vi "FTW_AppLauncher-Core_Process.vi"(0 "FTW Actor Instance Configuration":string="{\n  \"Identity\": \"ActorName\",\n  \"InboxAddress\": \"inproc://*\",\n  \"LoggerAddress\": \"\",\n  \"DebugEnableInboxLogging\": false,\n  \"DebugEnableJobLogging\": false,\n  \"LauncherAddress\": \"\",\n  \"My Data\": false,\n  \"Publisher URI\": \"inproc://*\",\n  \"Subscriber URIs\": \"\",\n  \"Refresh Period\": 2\n}", 11 "ErrorIn":errorcluster) -> (15 "Error":errorcluster)   [LabVIEW 2013, in "FTW-AppLauncher-Core.lvclass"]
uses:
  FTW-AppLauncher-Core.lvclass
  source/actor/Message/Base/FTW-Message.lvclass
  FTW-AppLauncher-Core.lvclass/FTW-AppLauncher-Core.ctl
  source/actor/Instance/FTW-ActorInstance.lvclass/FTW-ActorInstance.ctl
  source/actor/JobSequencer/FTW-SEQ-Current.vi
  source/actor/Instance/FTW-ActorInstance.lvclass
  source/actor/Message/Request/FTW-Message-IncomingRequest.lvclass
panel:
  out "Status":string
  # "shows the border of the run-time window\nthe orange box will not show"
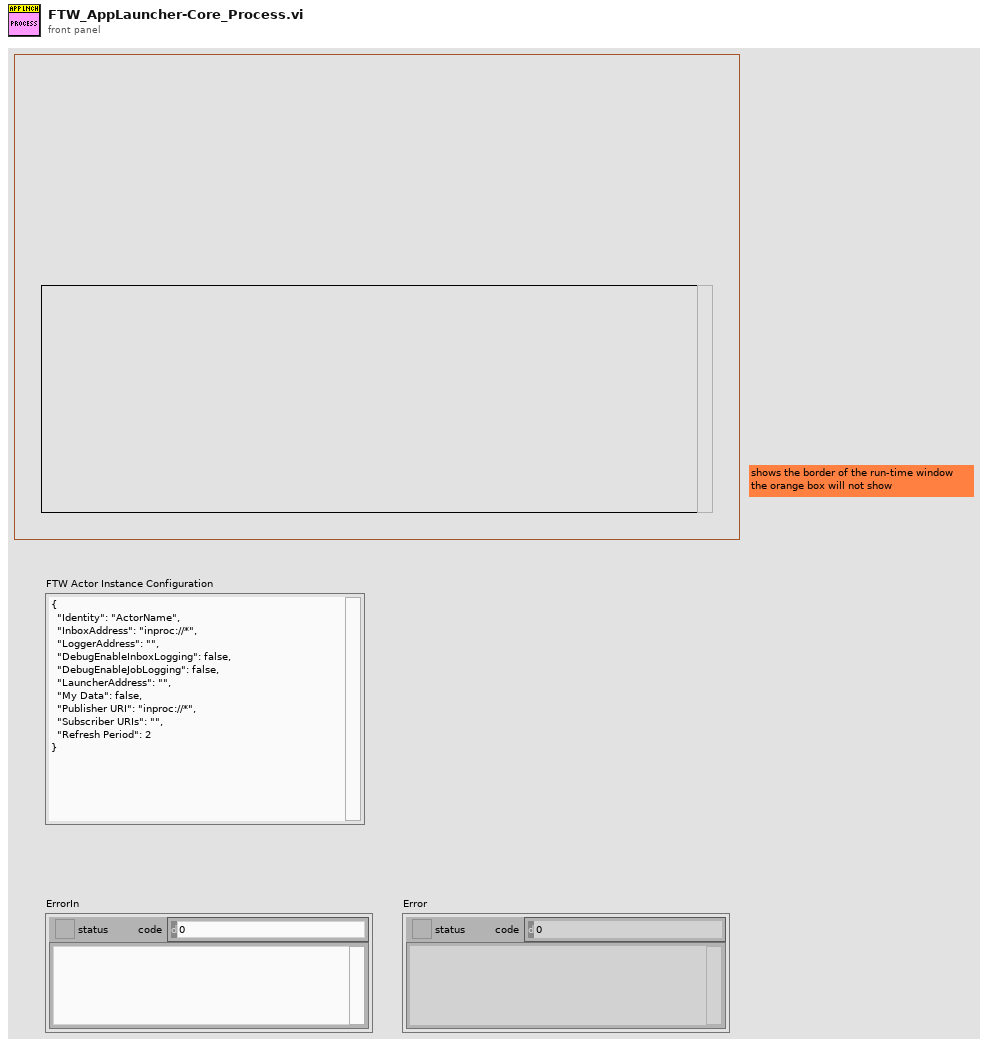
[diagram p1: front panel]
types:
  T1 = cluster{"Incoming Requests":refnum<event-registration>, "Local Messages":refnum<event-registration>, "Subscriber Registration":refnum<event-registration>}
  T2 = cluster{"Identity":string, "Instance Inbox Address":string}
  T3 = cluster{"String":string, "LabVIEW String":string}
  T4 = cluster{"String":string, "LabVIEW String":string}[]
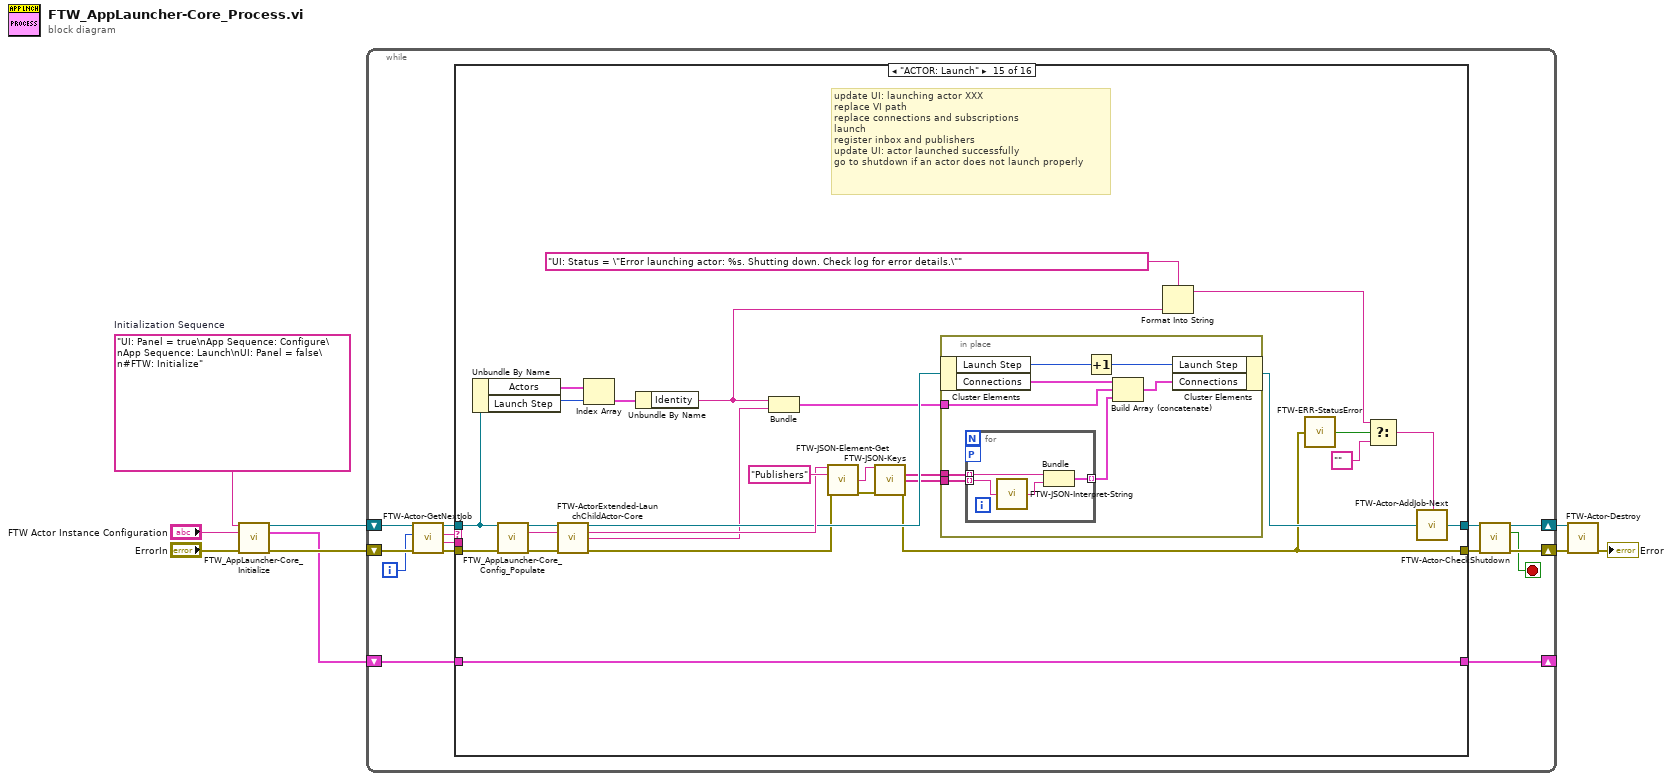
[diagram p0: block diagram]
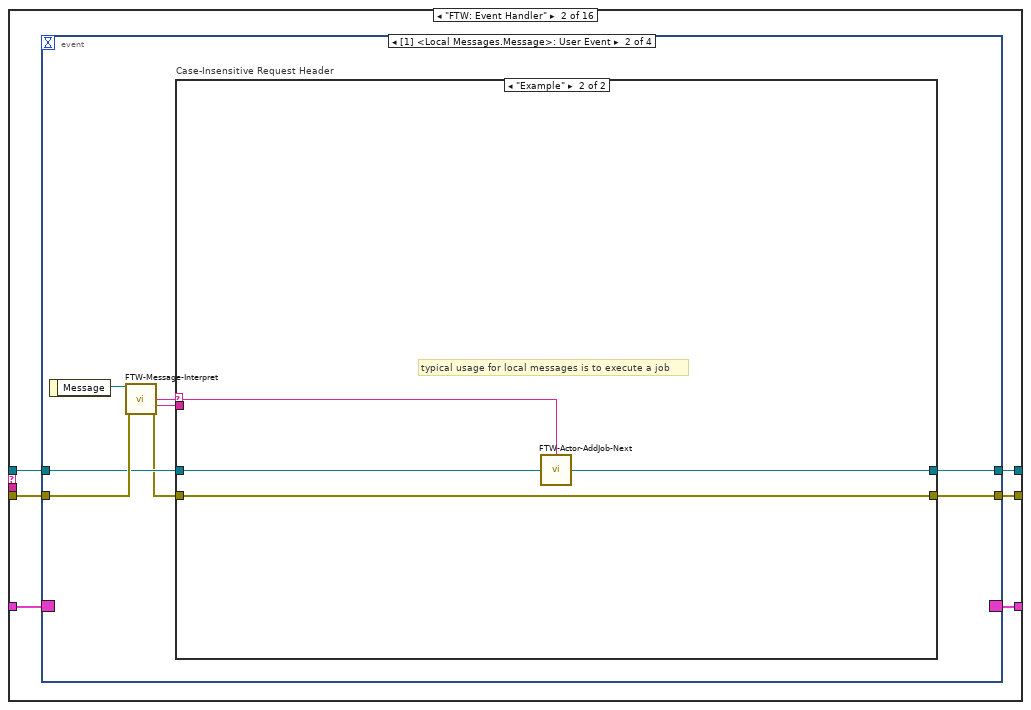
[diagram p3: hidden frame]
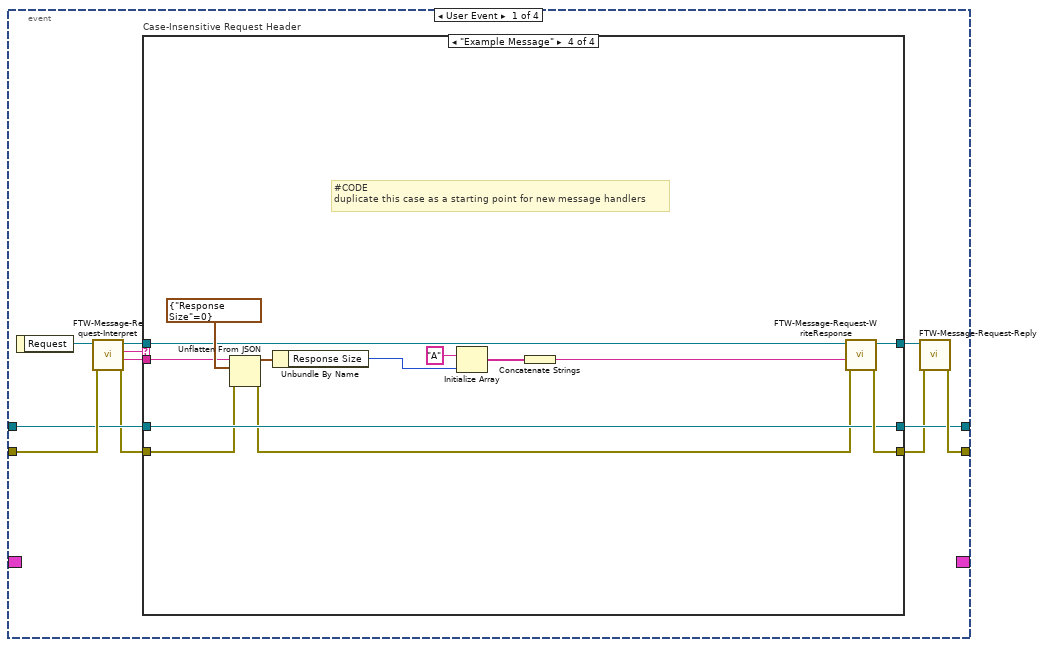
[diagram p4: hidden frame]
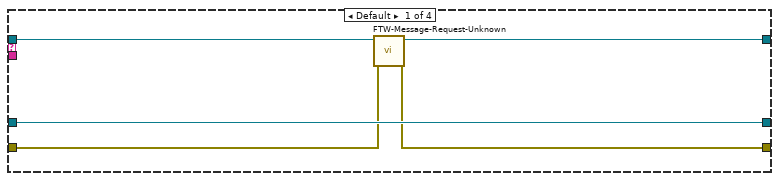
[diagram p5: hidden frame]
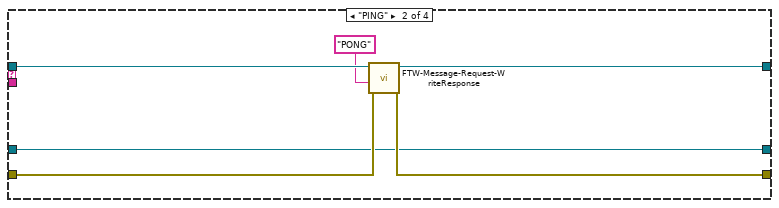
[diagram p6: hidden frame]
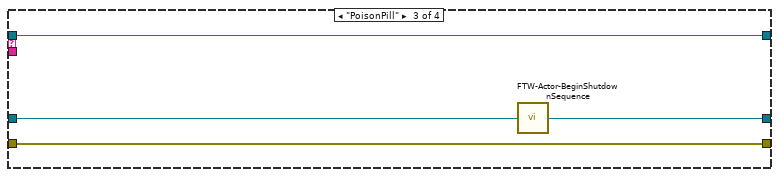
[diagram p7: hidden frame]
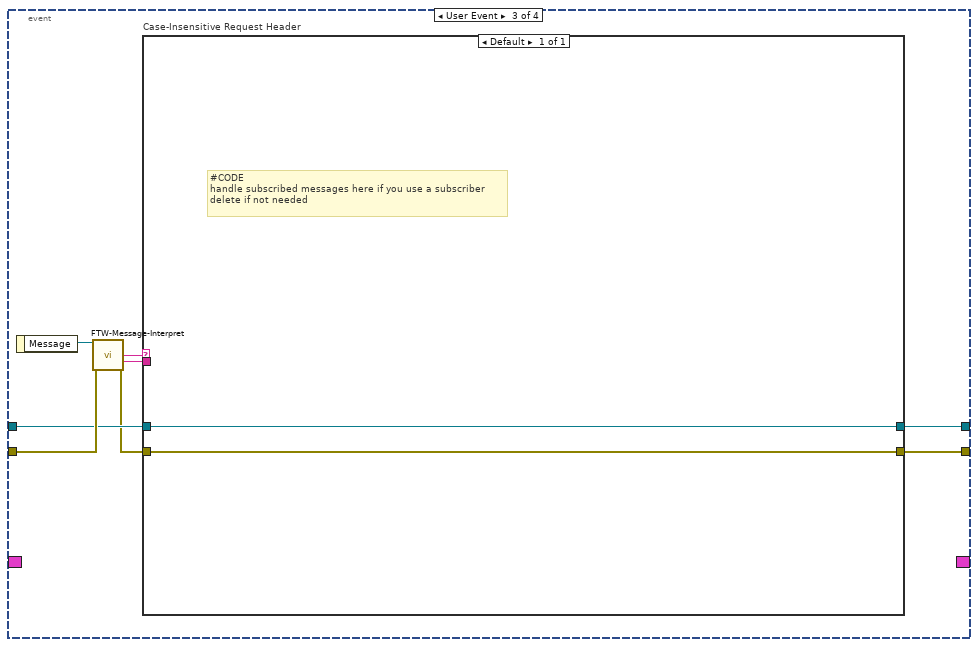
[diagram p9: hidden frame]
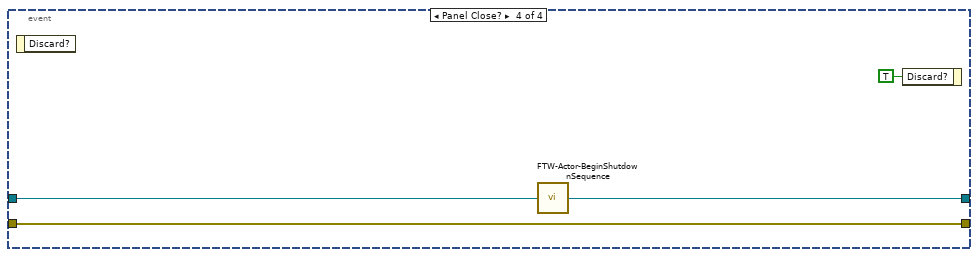
[diagram p10: hidden frame]
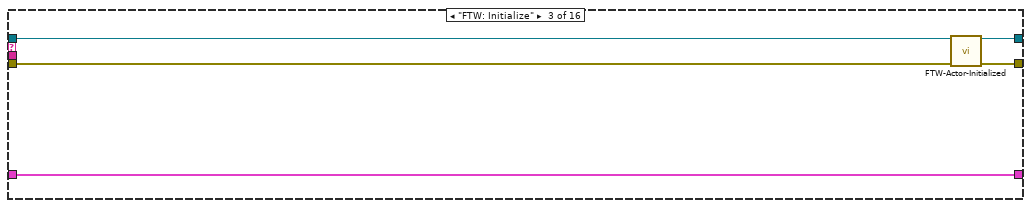
[diagram p11: hidden frame]
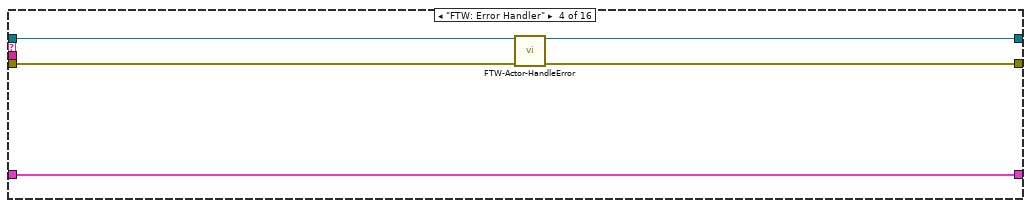
[diagram p12: hidden frame]
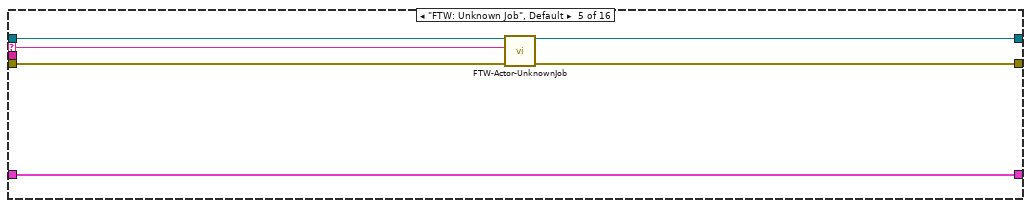
[diagram p13: hidden frame]
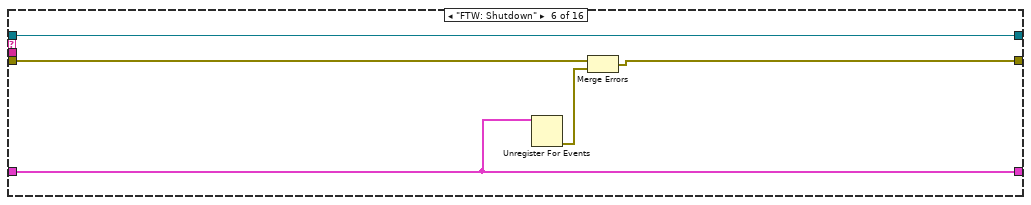
[diagram p14: hidden frame]
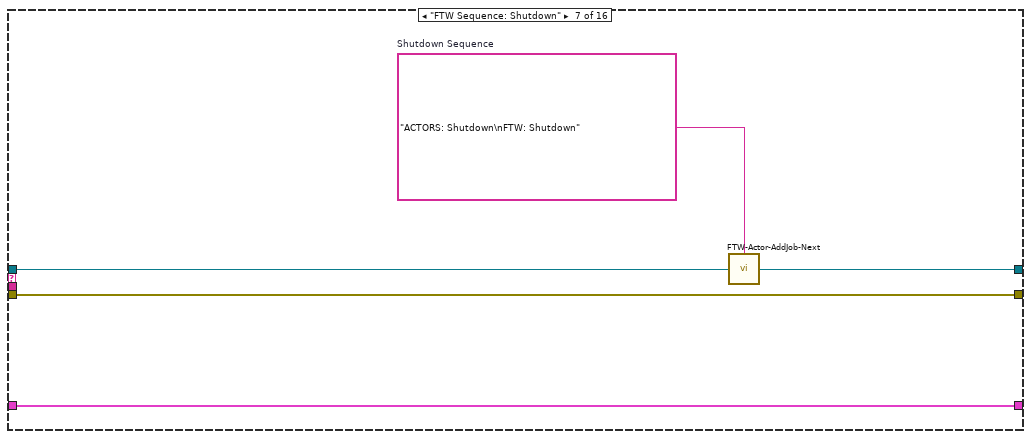
[diagram p15: hidden frame]
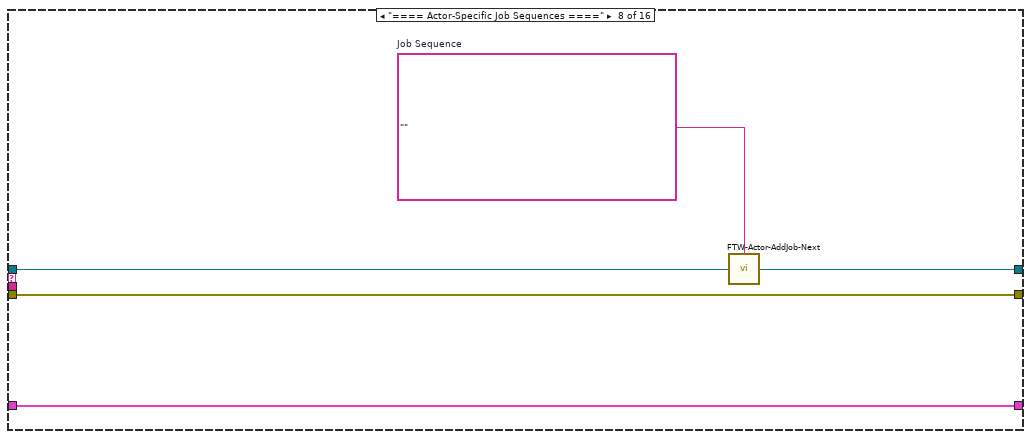
[diagram p16: hidden frame]
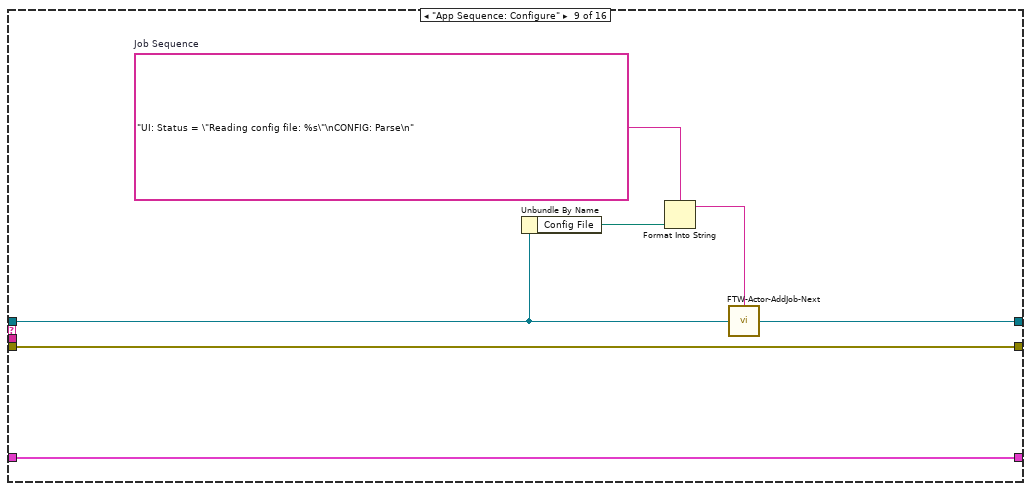
[diagram p17: hidden frame]
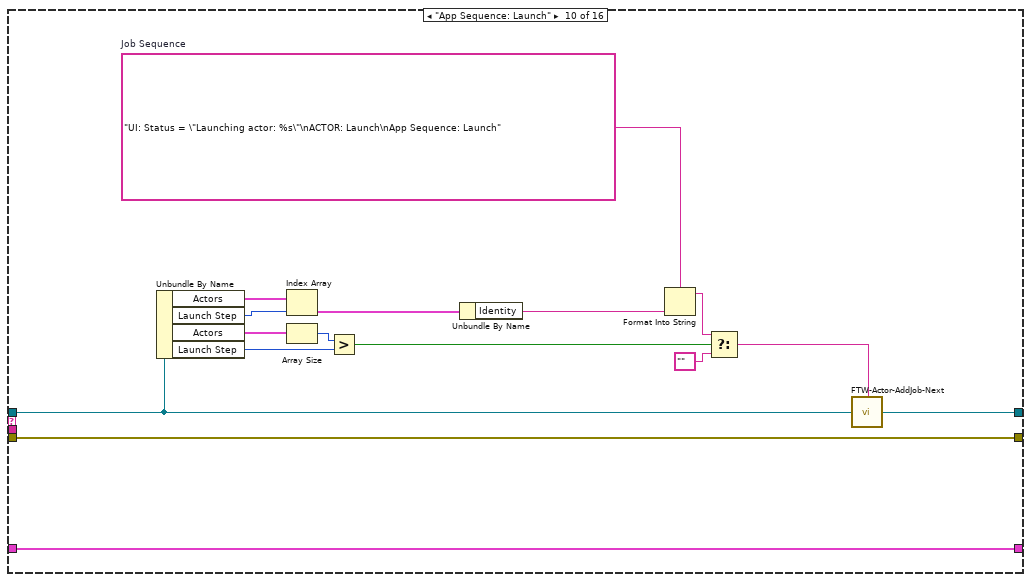
[diagram p18: hidden frame]
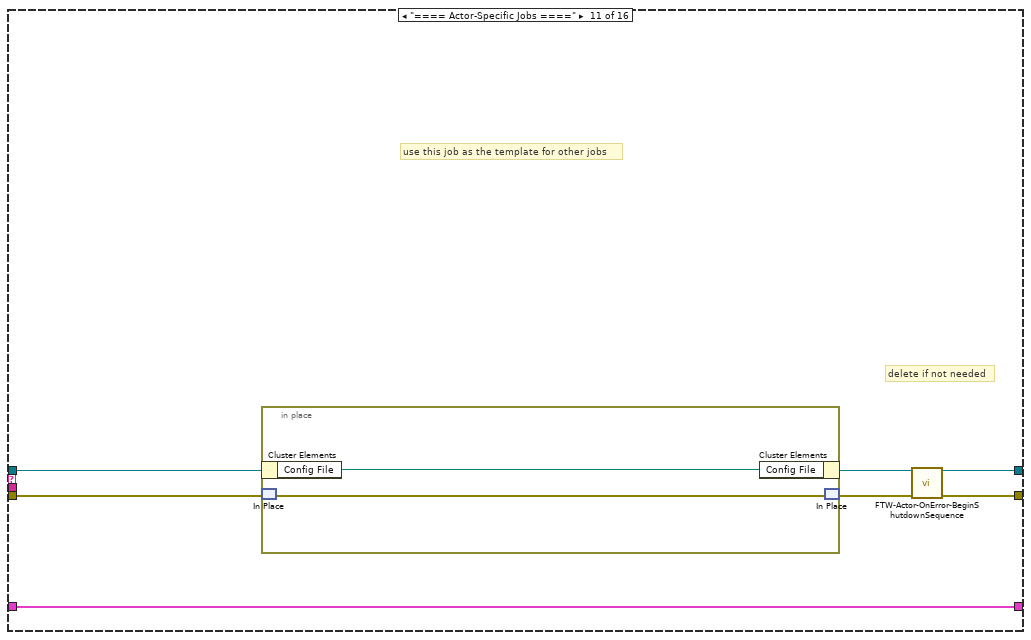
[diagram p19: hidden frame]
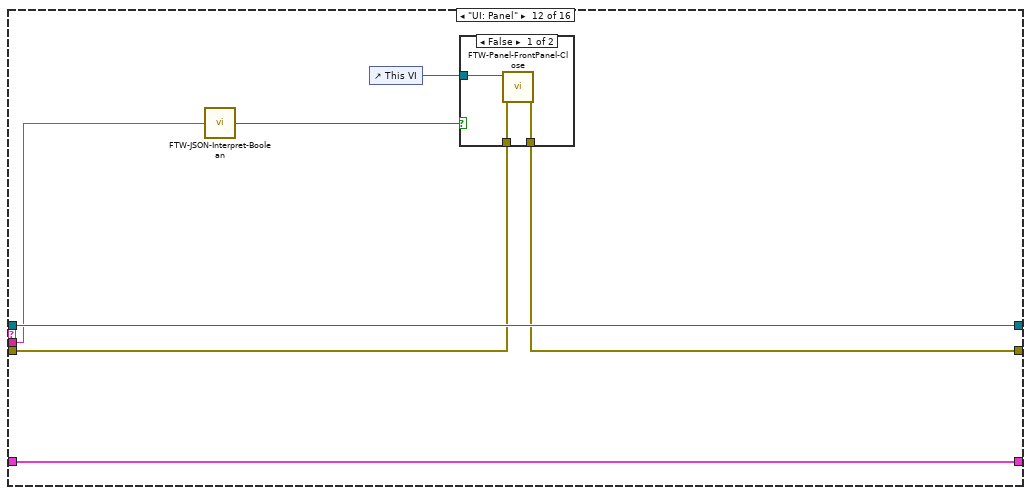
[diagram p20: hidden frame]
diagram:
  w5 = "UI: Panel = true\nApp Sequence: Configure\nApp Sequence: Launch\nUI: Panel = false\n#FTW: Initialize"  # Initialization Sequence
  n1 = call "FTW_AppLauncher-Core_Initialize.vi"("Initialization Sequence"=w5, "FTW Actor Instance Configuration"="FTW Actor Instance Configuration", "error in (no error)"="ErrorIn") -> ("Actor Template-Core out"=w1:refnum<class "FTW-AppLauncher-Core.lvclass">, "Event Refnums"=w2:T1, "error out"=w6:errorcluster)  [unwired: 9 in, 1 out]
  n2 = while {
    shift-right: [w13] -> w8
    shift-left: w6 -> [w20]
    shift-right: [w10] -> _
    shift-left: w2 -> [w23]
    shift-right: [w15] -> w9
    shift-left: w1 -> [w22]
    i -> [w11]
    stop <- w12 stop-if-true
    n3 = call "FTW-Actor-GetNextJob.vi"("error in"=w20, "Jobs Performed"=w11, "FTW Actor Instance"=w22) -> ("error out"=w19:errorcluster, "Job Data"=w17:string, "Job Name"=w18:string, "FTW Actor Instance out"=w21:refnum<class "FTW-AppLauncher-Core.lvclass">)  [unwired: 5 in]
    n4 = case shown="\"ACTOR: Launch\"" w18 {
      selector: w18 -> [_ _ _ _ w110 _ _ _ _ _ _ _ _ _ _ _]
      tunnel: [w25 w32 w101 w106 w113 w119 w124 w129 w136 w152 w156 w165 w189 w195 w211 w250] -> w14
      tunnel: w19 -> [w25 w31 w103 w108 w114 w120 w124 w129 w136 w152 w159 w166 w193 w204 w235 w251]
      tunnel: w23 -> [w26 w27 w104 w109 w115 w117 w125 w130 w137 w153 w160 w169 w194 w205 w236 w253]
      tunnel: [w26 w30 w104 w109 w115 w117 w125 w130 w137 w153 w160 w169 w194 w205 w236 w253] -> w10
      tunnel: w17 -> [_ _ _ _ _ _ _ _ _ _ _ w164 w190 _ _ _]
      tunnel: [w24 w29 w102 w107 w111 w116 w122 w127 w135 w151 w154 w168 w187 w196 w214 w252] -> w16
      tunnel: w21 -> [w24 w28 w100 w105 w112 w116 w123 w128 w132 w149 w157 w168 w188 w203 w220 w252]
      frame "==== Featherweight Framework Jobs ====" {
      }
      frame "FTW: Event Handler" {
        n5 = event shown="[1] <Local Messages.Message>: User Event" {
          selector: w27 -> [_ _ _ _]
          dyn-events: [_ _ _ _] -> w30
          timeout: _ -> [_ _ _ _]
          tunnel: [w42 w74 w88 w98] -> w32
          tunnel: w31 -> [w41 w78 w92 w98]
          tunnel: [w36 w75 w89 w96] -> w29
          tunnel: w28 -> [w40 w77 w91 w97]
          event User Event {
            n6 = event-data() -> ("Request"=w43:refnum<class "FTW-Message-IncomingRequest.lvclass">)  [unwired: 1 in]
            n7 = call "FTW-Message-Request-Interpret.vi"("error in"=w41, "FTW Incoming Request"=w43) -> ("error out"=w39:errorcluster, "Request Body"=w33:string, "Request Header"=w37:string, "FTW Incoming Request out"=w38:refnum<class "FTW-Message-IncomingRequest.lvclass">)  [unwired: 6 in]
            n8 = case "Case-Insensitive Request Header" shown="\"Example Message\"" w37 {
              tunnel: [w46 w52 w57 w71] -> w35
              tunnel: w39 -> [w47 w53 w57 w60]
              tunnel: [w48 w51 w58 w69] -> w36
              tunnel: w40 -> [w48 w51 w56 w69]
              tunnel: w38 -> [w45 w54 w55 w61]
              tunnel: [w44 w50 w55 w70] -> w34
              tunnel: w33 -> [_ _ _ w59]
              frame Default {
                n9 = call "FTW-Message-Request-Unknown.vi"("error in"=w47, "FTW Incoming Request"=w45) -> ("error out"=w46:errorcluster, "FTW Incoming Request Out"=w44:refnum<class "FTW-Message-IncomingRequest.lvclass">)  [unwired: 8 in]
              }
              frame "PING" {
                n10 = call "FTW-Message-Request-WriteResponse.vi"("error in"=w53, "Response Body"="PONG" ("Response Header"), "FTW Incoming Request"=w54) -> ("error out"=w52:errorcluster, "FTW Incoming Request out"=w50:refnum<class "FTW-Message-IncomingRequest.lvclass">)  [unwired: 7 in]
              }
              frame "PoisonPill" {
                n11 = call "FTW-Actor-BeginShutdownSequence.vi"("FTW Actor Instance"=w56) -> ("FTW Actor Instance out"=w58:refnum<class "FTW-AppLauncher-Core.lvclass">)  [unwired: 3 in]
              }
              frame "Example Message" {
                # "#CODE\nduplicate this case as a starting point for new message handlers"
                n12 = Unflatten From JSON(JSON string=w59, type and defaults=cluster{"Response Size":i32} {"Response Size"=0}, error in (no error)=w60) -> (value=w66:cluster{"Response Size":i32}, error out=w68:errorcluster)  [unwired: 4 in]
                n13 = Unbundle By Name(w66) -> ("Response Size"=w65:i32)
                n14 = Initialize Array("A", w65) -> (w63:string[])
                n15 = Concatenate Strings(w63) -> (w62:string)
                n16 = call "FTW-Message-Request-WriteResponse.vi"("error in"=w68, "Response Body"=w62, "FTW Incoming Request"=w61) -> ("error out"=w71:errorcluster, "FTW Incoming Request out"=w70:refnum<class "FTW-Message-IncomingRequest.lvclass">)  [unwired: 7 in]
              }
            }
            n17 = call "FTW-Message-Request-Reply.vi"("FTW: Reply Error"=w35, "FTW Incoming Request"=w34) -> ("error out"=w42:errorcluster)  [unwired: 8 in, 1 out]
          }
          event User Event {
            n18 = event-data() -> ("Message"=w79:refnum<class "FTW-Message.lvclass">)  [unwired: 1 in]
            n19 = call-dynamic "FTW-Message-Interpret.vi"("FTW Message"=w79, "error in"=w78) -> ("Message Header"=w73:string, "Message Body"=w72:string, "error out"=w76:errorcluster)  [unwired: 9 in, 2 out]
            n20 = case "Case-Insensitive Request Header" shown="\"Example\"" w73 {
              selector: w73 -> [_ w82]
              tunnel: [w80 w84] -> w74
              tunnel: w76 -> [w80 w84]
              tunnel: [w81 w83] -> w75
              tunnel: w77 -> [w81 w85]
              tunnel: w72 -> [_ _]
              frame Default {
                # "#CODE\nhandle local messages here\ndelete if not needed"
              }
              frame "Example" {
                # "typical usage for local messages is to execute a job"
                n21 = call "FTW-Actor-AddJob-Next.vi"("Add Next in Job Queue"=w82, "FTW Actor Instance"=w85) -> ("FTW Actor Instance out"=w83:refnum<class "FTW-AppLauncher-Core.lvclass">)  [unwired: 2 in]
              }
            }
          }
          event User Event {
            n22 = event-data() -> ("Message"=w93:refnum<class "FTW-Message.lvclass">)  [unwired: 1 in]
            n23 = call-dynamic "FTW-Message-Interpret.vi"("FTW Message"=w93, "error in"=w92) -> ("Message Header"=w87:string, "Message Body"=w86:string, "error out"=w90:errorcluster)  [unwired: 9 in, 2 out]
            n24 = case "Case-Insensitive Request Header" shown="Default" w87 {
              tunnel: [w94] -> w88
              tunnel: w90 -> [w94]
              tunnel: [w95] -> w89
              tunnel: w91 -> [w95]
              tunnel: w86 -> [_]
              frame Default {
                # "#CODE\nhandle subscribed messages here if you use a subscriber\ndelete if not needed"
              }
            }
          }
          event Panel Close? {
            n25 = event-data() -> ()  [unwired: 1 in, 1 out]
            n26 = call "FTW-Actor-BeginShutdownSequence.vi"("FTW Actor Instance"=w97) -> ("FTW Actor Instance out"=w96:refnum<class "FTW-AppLauncher-Core.lvclass">)  [unwired: 3 in]
            n27 = event-data("Discard?"=TRUE) -> ()  [unwired: 1 in, 1 out]
          }
        }
      }
      frame "FTW: Initialize" {
        n28 = call-dynamic "FTW-Actor-Initialized.vi"("FTW Actor Instance"=w100, "error in"=w103) -> ("FTW Actor Instance out"=w102:refnum<class "FTW-AppLauncher-Core.lvclass">, "error out"=w101:errorcluster)  [unwired: 12 in]
      }
      frame "FTW: Error Handler" {
        n29 = call-dynamic "FTW-Actor-HandleError.vi"("FTW Actor Instance"=w105, "error in"=w108) -> ("FTW Actor Instance out"=w107:refnum<class "FTW-AppLauncher-Core.lvclass">, "error out"=w106:errorcluster)  [unwired: 10 in, 2 out]
      }
      frame "FTW: Unknown Job", Default {
        n30 = call-dynamic "FTW-Actor-UnknownJob.vi"("FTW Actor Instance"=w112, "Unknown Job"=w110, "error in"=w114) -> ("FTW Actor Instance out"=w111:refnum<class "FTW-AppLauncher-Core.lvclass">, "error out"=w113:errorcluster)  [unwired: 11 in]
      }
      frame "FTW: Shutdown" {
        n31 = Unregister For Events(event registration refnum=w117) -> (error out=w118:errorcluster)  [unwired: 1 in]
        n32 = Merge Errors(w120, w118) -> (w119:errorcluster)
      }
      frame "FTW Sequence: Shutdown" {
        w121 = "ACTORS: Shutdown\nFTW: Shutdown"  # Shutdown Sequence
        n33 = call "FTW-Actor-AddJob-Next.vi"("Add Next in Job Queue"=w121, "FTW Actor Instance"=w123) -> ("FTW Actor Instance out"=w122:refnum<class "FTW-AppLauncher-Core.lvclass">)  [unwired: 2 in]
      }
      frame "==== Actor-Specific Job Sequences ====" {
        w126 = ""  # Job Sequence
        n34 = call "FTW-Actor-AddJob-Next.vi"("Add Next in Job Queue"=w126, "FTW Actor Instance"=w128) -> ("FTW Actor Instance out"=w127:refnum<class "FTW-AppLauncher-Core.lvclass">)  [unwired: 2 in]
      }
      frame "App Sequence: Configure" {
        w134 = "UI: Status = \"Reading config file: %s\"\nCONFIG: Parse\n"  # Job Sequence
        n35 = Unbundle By Name(w132) -> ("Config File"=w131:path)
        n36 = Format Into String(format string=w134, w131) -> (resulting string=w133:string)  [unwired: 2 in, 1 out]
        n37 = call "FTW-Actor-AddJob-Next.vi"("Add Next in Job Queue"=w133, "FTW Actor Instance"=w132) -> ("FTW Actor Instance out"=w135:refnum<class "FTW-AppLauncher-Core.lvclass">)  [unwired: 2 in]
      }
      frame "App Sequence: Launch" {
        w150 = "UI: Status = \"Launching actor: %s\"\nACTOR: Launch\nApp Sequence: Launch"  # Job Sequence
        n38 = Unbundle By Name(w149) -> ("Actors"=w141:cluster{"Identity":string, "Config":string}[], "Launch Step"=w140:i32, "Actors"=w148:cluster{"Identity":string, "Config":string}[], "Launch Step"=w146:i32)
        n39 = Index Array(array=w141, index=w140) -> (element=w139:cluster{"Identity":string, "Config":string})
        n40 = Array Size(array=w148) -> (size(s)=w147:i32)
        n41 = Greater?(x=w147, y=w146) -> (0:w144:bool)
        n42 = Unbundle By Name(w139) -> ("Identity"=w138:string)
        n43 = Format Into String(format string=w150, w138) -> (resulting string=w145:string)  [unwired: 2 in, 1 out]
        n44 = Select(t=w145, s=w144, f="" ("empty string")) -> (s? t:f=w143:string)
        n45 = call "FTW-Actor-AddJob-Next.vi"("Add Next in Job Queue"=w143, "FTW Actor Instance"=w149) -> ("FTW Actor Instance out"=w151:refnum<class "FTW-AppLauncher-Core.lvclass">)  [unwired: 2 in]
      }
      frame "==== Actor-Specific Jobs ====" {
        # "delete if not needed"
        # "use this job as the template for other jobs"
        n46 = in-place {
          n47 = in-place-cluster #1(w157) -> ("Config File"=w161:path)
          n48 = in-place-match #2(w159) -> (w162:errorcluster)
          n49 = in-place-cluster #1("Config File"=w161) -> (w155:refnum<class "FTW-AppLauncher-Core.lvclass">)
          n50 = in-place-match #2(w162) -> (w158:errorcluster)
        }
        n51 = call-dynamic "FTW-Actor-OnError-BeginShutdownSequence.vi"("FTW Actor Instance"=w155, "error in"=w158) -> ("FTW Actor Instance out"=w154:refnum<class "FTW-AppLauncher-Core.lvclass">, "error out"=w156:errorcluster)  [unwired: 12 in]
      }
      frame "UI: Panel" {
        n52 = call "FTW-JSON-Interpret-Boolean.vi"("JSON Boolean"=w164) -> ("LabVIEW Boolean"=w163:bool)
        n53 = control-ref of="This VI"() -> (w167:refnum<vi>)
        n54 = case shown="False" w163 {
          tunnel: w167 -> [w172 w173]
          tunnel: w166 -> [w171 w175]
          tunnel: [w170 w174] -> w165
          frame False {
            n55 = call "FTW-Panel-FrontPanel-Close.vi"("error in"=w171, "VI Ref"=w172) -> ("error out"=w170:errorcluster)  [unwired: 8 in, 1 out]
          }
          frame True {
            n56 = call "FTW-Panel-FrontPanel-Open.vi"("error in"=w175, "VI Ref"=w173) -> ("error out"=w174:errorcluster)  [unwired: 8 in, 1 out]
          }
        }
      }
      frame "UI: Status" {
        n57 = Get Date/Time In Seconds() -> (seconds since 1Jan1904=w179:timestamp)
        n58 = call "FTW-JSON-Interpret-String.vi"("JSON String"=w190) -> ("LabVIEW String"=w185:string)
        n59 = feedback #3(w179) -> (w180:timestamp)
        n60 = feedback-in #3(w180) -> ()
        n61 = Subtract(x=w179, y=w180) -> (x-y=w178:dbl)
        n62 = call-dynamic "FTW-Actor-Log-Event.vi"("FTW Actor Instance"=w188, "Event Type"="Launching", "Event Data"=w185, "Source (unwired for identity)"="" ("empty string"), "error in"=w193) -> ("FTW Actor Instance out"=w187:refnum<class "FTW-AppLauncher-Core.lvclass">, "Serialized Event"=w183:string, "error out"=w189:errorcluster)  [unwired: 8 in]
        n63 = Format Into String(format string="[%06.3fsec]", w178) -> (resulting string=w176:string)  [unwired: 2 in, 1 out]
        n64 = local read "Status"() -> (w192:string)
        n65 = Concatenate Strings(w192, "\r", w176, w183) -> (w182:string)
        n66 = property on="Status" class="Str"("Value"=w182, "Text.Scroll Position"=u32 4294967295) -> ()  [unwired: 2 in, 2 out]
      }
      frame "CONFIG: Parse" {
        n67 = Unbundle By Name(w203) -> ("Config File"=w201:path)
        n68 = Read from Text File(file (use dialog)=w201, error in=w204) -> (text=w200:string, error out=w202:errorcluster)  [unwired: 2 in, 2 out]
        n69 = call "FTW_AppLauncher-Core_Config_Parse.vi"("Config String"=w200, "error in"=w202) -> ("Actors"=w199:string[], "Configurations"=w198:string[], "error out"=w195:errorcluster)  [unwired: 11 in]
        n70 = for {
          tunnel: w199 -> [w208] mode=indexing
          tunnel: w198 -> [w207] mode=indexing
          tunnel: [w206] -> w197 mode=indexing
          workers-P: _ -> [_]
          n71 = Bundle("String"=w208, "String"=w207) -> (w206:cluster{"String":string, "String":string})  [unwired: 1 in]
        }
        n72 = Bundle By Name(cluster=w203, "Actors"=w197) -> (w196:refnum<class "FTW-AppLauncher-Core.lvclass">)
      }
      frame "ACTOR: Launch" {
        # "update UI: launching actor XXX\nreplace VI path\nreplace connections and subscriptions\nlaunch\nregister inbox and publishers\nupdate UI: actor launched successfully\ngo to shutdown if an actor does not launch properly"
        n73 = Unbundle By Name(w220) -> ("Actors"=w219:cluster{"Identity":string, "Config":string}[], "Launch Step"=w218:i32)
        n74 = call "FTW_AppLauncher-Core_Config_Populate.vi"("FTW-AppLauncher-Core In"=w220, "error in"=w235) -> ("FTW-AppLauncher-Core Out"=w233:refnum<class "FTW-AppLauncher-Core.lvclass">, "Configuration String"=w232:string, "error out"=w234:errorcluster)  [unwired: 11 in]
        n75 = call-dynamic "FTW-ActorExtended-LaunchChildActor-Core.vi"("FTW Actor Instance Type"=w233, "Actor Instance Configuration"=w232, "error in"=w234) -> ("FTW Actor Instance"=w227:refnum<class "FTW-AppLauncher-Core.lvclass">, "Initialized Response"=w230:string, "Instance Inbox Address"=w223:string, "error out"=w221:errorcluster)  [unwired: 9 in]
        n76 = Index Array(array=w219, index=w218) -> (element=w217:cluster{"Identity":string, "Config":string})
        n77 = Unbundle By Name(w217) -> ("Identity"=w215:string)
        n78 = Bundle("Identity"=w215, "Instance Inbox Address"=w223) -> (w222:T2)  [unwired: 1 in]
        n79 = call "FTW-JSON-Element-Get.vi"("JSON Opject"=w230, "Key"="Publishers", "error in"=w221) -> ("Element"=w229:string, "error out"=w228:errorcluster)  [unwired: 10 in, 1 out]
        n80 = call "FTW-JSON-Keys.vi"("JSON Opject"=w229, "error in"=w228) -> ("Keys"=w225:string[], "Values"=w224:string[], "error out"=w211:errorcluster)  [unwired: 11 in]
        n81 = in-place {
          in-place-border: w225 -> [w244]
          in-place-border: w224 -> [w243]
          in-place-border: w222 -> [w240]
          n82 = in-place-cluster #4(w227) -> ("Launch Step"=w238:i32, "Connections"=w242:cluster{"Name":string, "Address":string}[])
          n83 = for {
            tunnel: w244 -> [w248] mode=indexing
            tunnel: w243 -> [w247] mode=indexing
            tunnel: [w245] -> w239 mode=indexing
            workers-P: _ -> [_]
            n84 = call "FTW-JSON-Interpret-String.vi"("JSON String"=w247) -> ("LabVIEW String"=w246:string)
            n85 = Bundle("String"=w248, "LabVIEW String"=w246) -> (w245:T3)  [unwired: 1 in]
          }
          n86 = Increment(x=w238) -> (x+1=w237:i32)
          n87 = Build Array (concatenate)(w242, w240, w239) -> (w241:T4)
          n88 = in-place-cluster #4("Launch Step"=w237, "Connections"=w241) -> (w226:refnum<class "FTW-AppLauncher-Core.lvclass">)
        }
        n89 = Format Into String(format string="UI: Status = \"Error launching actor: %s. Shutting down. Check log for error details.\"", w215) -> (resulting string=w213:string)  [unwired: 2 in, 1 out]
        n90 = call "FTW-ERR-StatusError.vi"("error to check"=w211) -> ("Error?"=w210:bool)
        n91 = Select(t=w213, s=w210, f="" ("empty string")) -> (s? t:f=w209:string)
        n92 = call "FTW-Actor-AddJob-Next.vi"("Add Next in Job Queue"=w209, "FTW Actor Instance"=w226) -> ("FTW Actor Instance out"=w214:refnum<class "FTW-AppLauncher-Core.lvclass">)  [unwired: 2 in]
      }
      frame "ACTORS: Static Links" {
        # "#TODO\nreplace with your actor"
        # "this case should never be executed\nit is here to statically link all your actors\nactors should inherit from the extended actor instance or pass back publisher addresses manually"
        n93 = vi-ref "FTW-ExtendedActorTemplate.vi"() -> ()  [unwired: 1 out]
        n94 = vi-ref "FTW-ExtendedActorTemplate.vi"() -> ()  [unwired: 1 out]
        n95 = vi-ref "FTW-ExtendedActorTemplate.vi"() -> ()  [unwired: 1 out]
        n96 = call "FTW-ERR-ThrowImpossibleError.vi"("Reason this error should never happen"="The static links job should never be executed. It is for linking only.", "error in"=w251) -> ("error out"=w250:errorcluster)  [unwired: 13 in]
        n97 = vi-ref "FTW-ExtendedActorTemplate.vi"() -> ()  [unwired: 1 out]
      }
    }
    n98 = call "FTW-Actor-CheckShutdown.vi"("FTW Actor Instance"=w16, "error in"=w14) -> ("FTW Actor Instance out"=w15:refnum<class "FTW-AppLauncher-Core.lvclass">, "Shutdown?"=w12:bool, "error out"=w13:errorcluster)  [unwired: 11 in]
  }
  n99 = call-dynamic "FTW-Actor-Destroy.vi"("FTW Actor Instance"=w9, "error in"=w8) -> ("error out"=→"Error":errorcluster)  [unwired: 13 in]
